vi "MDPtr Process Example.vi"() -> ()   [LabVIEW 2014]
uses:
  MDPtr TypeDef/MDPtr SupportedDataTypeDef.ctl
  _PolymorphicVIs/MDPtr Pack DoubleArr.vi
  _PolymorphicVIs/MDPtr Unpack DoubleArr.vi
panel:
  out "String Attribute":string
  out "MDPtr Total Count":i64
  out "FlattenStrPtr":string
  out "Copy Count":i32
  out "Data Type":T1
  out "error out":errorcluster
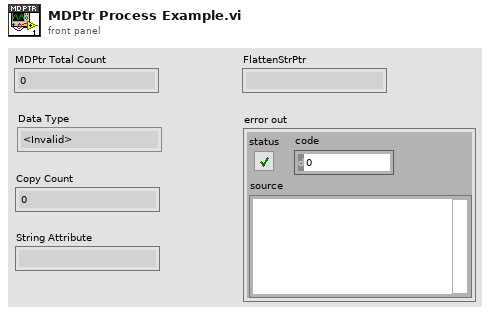
[diagram p1: front panel]
types:
  T1 = typedef "MDPtr SupportedDataTypeDef.ctl" = enum16{"<Invalid>", "Waveform", "Waveform Arr", "Double Arr", "String Arr"}
  T2 = typedef "MDPtr.ctl" = refnum<k1>
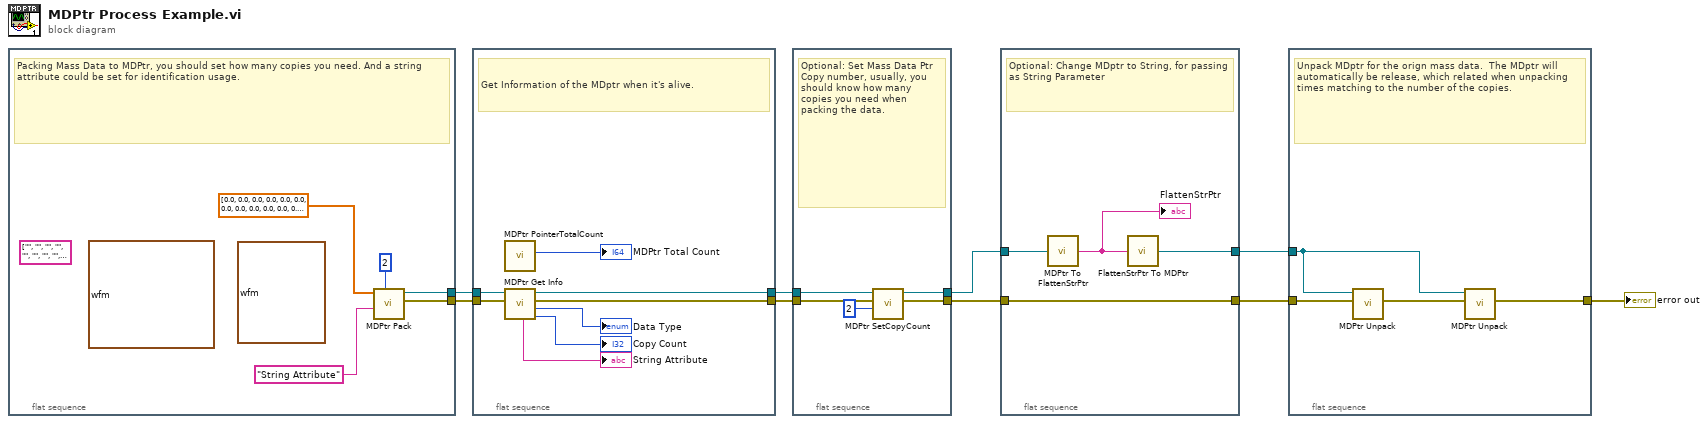
[diagram p0: block diagram]
diagram:
  n1 = flat-sequence {
    tunnel: [w14] -> w9
    tunnel: [w13] -> w8
    frame #0 {
      (unwired) string[] ["", "", "", "", "", "", "", "", "", "", "", "", "", "", "", "", "", "", "", "", "", "", "", "", "", "", "", "", "", "", "", "", "", "", "", "", "", "", "", "", "", "", "", "", "", "", "", "", "", "", "", "", "", "", "", "", "", "", "", "", "", "", "", "", "", "", "", "", "", "", "", "", "", "", "", "", "", "", "", "", "", "", "", "", "", "", "", "", "", "", "", "", "", "", "", "", "", "", "", "", "", "", "", "", "", "", "", "", "", "", "", "", "", "", "", "", "", "", "", "", "", "", "", "", "", "", "", "", "", "", "", "", "", "", "", "", "", "", "", "", "", "", "", "", "", "", "", "", "", "", "", "", "", "", "", "", "", "", "", "", "", "", "", "", "", "", "", "", "", "", "", "", "", "", "", "", "", "", "", "", "", "", "", "", "", "", "", "", "", "", "", "", "", "", "", "", "", "", "", "", ""] ("Y")
      (unwired) waveform(dbl) {"t0"=timestamp(0 s since 1904-01-01), "dt"=1.0, "Y"=[]} ("waveform")
      (unwired) waveform(dbl)[] [{"t0"=timestamp(0 s since 1904-01-01), "dt"=1.0, "Y"=[]}, {"t0"=timestamp(0 s since 1904-01-01), "dt"=2.0, "Y"=[]}] ("waveforms")
      # "Packing Mass Data to MDPtr, you should set how many copies you need. And a string attribute could be set for identification usage."
      n2 = call-poly "MDPtr Pack.vi"("Copies Count(1)"=2, "String Attribute"="String Attribute", "Double Array"=dbl[] [0.0, 0.0, 0.0, 0.0, 0.0, 0.0, 0.0, 0.0, 0.0, 0.0, 0.0, 0.0, 0.0, 0.0, 0.0, 0.0, 0.0, 0.0, 0.0, 0.0, 0.0, 0.0, 0.0, 0.0, 0.0, 0.0, 0.0, 0.0, 0.0, 0.0, 0.0, 0.0, 0.0, 0.0, 0.0, 0.0, 0.0, 0.0, 0.0, 0.0, 0.0, 0.0, 0.0, 0.0, 0.0, 0.0, 0.0, 0.0, 0.0, 0.0, 0.0, 0.0, 0.0, 0.0, 0.0, 0.0, 0.0, 0.0, 0.0, 0.0, 0.0, 0.0, 0.0, 0.0, 0.0, 0.0, 0.0, 0.0, 0.0, 0.0, 0.0, 0.0, 0.0, 0.0, 0.0, 0.0, 0.0, 0.0, 0.0, 0.0, 0.0, 0.0, 0.0, 0.0, 0.0, 0.0, 0.0, 0.0, 0.0, 0.0, 0.0, 0.0, 0.0, 0.0, 0.0, 0.0, 0.0, 0.0, 0.0, 0.0, 0.0, 0.0, 0.0, 0.0, 0.0, 0.0, 0.0, 0.0, 0.0, 0.0, 0.0, 0.0, 0.0, 0.0, 0.0, 0.0, 0.0, 0.0, 0.0, 0.0, 0.0, 0.0, 0.0, 0.0, 0.0, 0.0, 0.0, 0.0, 0.0, 0.0, 0.0, 0.0, 0.0, 0.0, 0.0, 0.0, 0.0, 0.0, 0.0, 0.0, 0.0, 0.0, 0.0, 0.0, 0.0, 0.0, 0.0, 0.0, 0.0, 0.0, 0.0, 0.0, 0.0, 0.0, 0.0, 0.0, 0.0, 0.0, 0.0, 0.0, 0.0, 0.0, 0.0, 0.0, 0.0, 0.0, 0.0, 0.0, 0.0, 0.0, 0.0, 0.0, 0.0, 0.0, 0.0, 0.0, 0.0, 0.0, 0.0, 0.0, 0.0, 0.0, 0.0, 0.0, 0.0, 0.0, 0.0, 0.0, 0.0, 0.0, 0.0, 0.0, 0.0, 0.0, 0.0, 0.0, 0.0, 0.0, 0.0, 0.0, 1.0] ("Y")) -> ("error out"=w13:errorcluster, "HexStrPtr"=w14:T2)  [unwired: 7 in]
    }
  }
  n3 = flat-sequence {
    tunnel: w9 -> [w22]
    tunnel: w8 -> [w21]
    tunnel: [w18] -> w7
    tunnel: [w17] -> w6
    frame #0 {
      # "Get Information of the MDptr when it's alive."
      n4 = call "MDPtr PointerTotalCount.vi"() -> ("MDPtr Total Count"=→"MDPtr Total Count":i64)  [unwired: 10 in, 1 out]
      n5 = call "MDPtr Get Info.vi"("error in (no error)"=w21, "HexStrPtr"=w22) -> ("Copy Count"=→"Copy Count":i32, "Data Type"=→"Data Type":T1, "error out"=w17:errorcluster, "HexStrPtr (dup)"=w18:T2, "String Attribute"=→"String Attribute":string)  [unwired: 5 in]
    }
  }
  n6 = flat-sequence {
    tunnel: w7 -> [w27]
    tunnel: w6 -> [w26]
    tunnel: [w24] -> w4
    tunnel: [w23] -> w1
    frame #0 {
      # "Optional: Set Mass Data Ptr Copy number, usually, you should know how many copies you need when packing the data."
      n7 = call "MDPtr SetCopyCount.vi"("Copy Count"=2, "error in (no error)"=w26, "HexStrPtr"=w27) -> ("error out"=w23:errorcluster, "HexStrPtr (dup)"=w24:T2)  [unwired: 6 in]
    }
  }
  n8 = flat-sequence {
    tunnel: w4 -> [w30]
    tunnel: [w29] -> w3
    tunnel: [w28] -> w2
    tunnel: w1 -> [w28]
    frame #0 {
      # "Optional: Change MDptr to String, for passing as String Parameter"
      n9 = call "MDPtr To FlattenStrPtr.vi"("HexStrPtr"=w30) -> ("FlattenStrPtr"=w31:string)
      "FlattenStrPtr" <- w31
      n10 = call "FlattenStrPtr To MDPtr.vi"("FlattenStrPtr"=w31) -> ("HexStrPtr"=w29:T2)
    }
  }
  n11 = flat-sequence {
    tunnel: [w34] -> w5
    tunnel: w3 -> [w33]
    tunnel: w2 -> [w32]
    frame #0 {
      # "Unpack MDptr for the orign mass data.  The MDptr will automatically be release, which related when unpacking times matching to the number of the copies."
      n12 = call-poly "MDPtr Unpack.vi"("error in (no error)"=w32, "HexStrPtr"=w33) -> ("error out"=w35:errorcluster)  [unwired: 7 in, 2 out]
      n13 = call-poly "MDPtr Unpack.vi"("error in (no error)"=w35, "HexStrPtr"=w33) -> ("error out"=w34:errorcluster)  [unwired: 7 in, 2 out]
    }
  }
  "error out" <- w5
